vi "CString vs LStr Performance Comparison.vi"() -> ()   [LabVIEW 2020]
uses:
  <vilib>/Utility/file.llb/Application Directory.vi
  <vilib>/Utility/libraryn.llb/Check if File or Folder Exists.vi
panel:
  out "LStr Lossy Time":dbl
  out "LStr Lossy Results":i32[](array[numeric])
  out "CString Results":i32[](array[numeric])
  out "LStr Results":i32[](array[numeric])
  out "LStr Time":dbl
  out "CString Time":dbl
  # "This compares the performance between CStrings and LStr.\n\nAs expected LStr performance is better since it is the internal format.\n\nThis is aided by the speed of the encoding library vs the lossy from utf8."
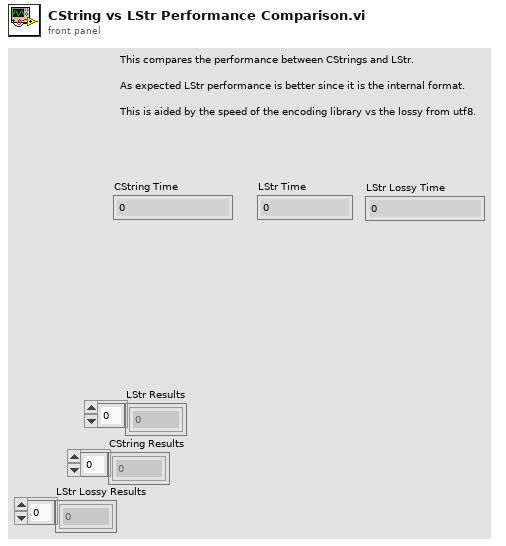
[diagram p1: front panel]
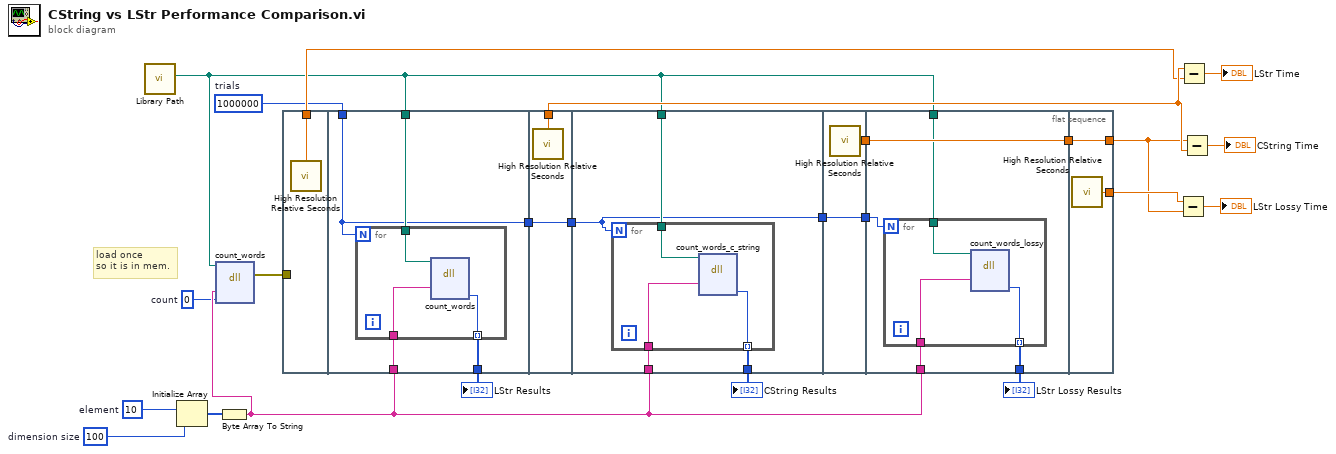
[diagram p0: block diagram]
diagram:
  w2 = 0  # count
  w14 = 100  # dimension size
  w15 = u8 10  # element
  w20 = 1000000  # trials
  # "load once\nso it is in mem."
  n1 = call "Library Path.vi"() -> ("Library Path"=w3:path)  [unwired: 11 in]
  n2 = Initialize Array(w15, w14) -> (w13:u8[])
  n3 = Byte Array To String(unsigned byte array=w13) -> (string=w4:string)
  n4 = dll-call lib="C:/Users/JamesMcNally/Documents/RustInterop/Rust-LabVIEW-Interop/target/debug/labview_test_library.dll" fn="count_words"(path in=w3, "string"=w4, "count"=w2) -> (error out=w1:errorcluster)  [unwired: 5 in, 1 out]
  n5 = flat-sequence {
    tunnel: [w25] -> w22
    tunnel: w1 -> [_]
    tunnel: w3 -> [w29]
    tunnel: w20 -> [w28]
    tunnel: [w28] -> w19
    tunnel: [w27] -> w17
    tunnel: w4 -> [w26]
    tunnel: [w34] -> w23
    tunnel: w19 -> [w33]
    tunnel: [w33] -> w18
    tunnel: w3 -> [w38]
    tunnel: w18 -> [w35]
    tunnel: [w37] -> w16
    tunnel: w4 -> [w36]
    tunnel: [w35] -> w6
    tunnel: [w43] -> w12
    tunnel: w6 -> [w42]
    tunnel: [w42] -> w5
    tunnel: w12 -> [w48]
    tunnel: w4 -> [w47]
    tunnel: w3 -> [w46]
    tunnel: [w45] -> w11
    tunnel: [w48] -> w10
    tunnel: w5 -> [w44]
    tunnel: [w53] -> w7
    tunnel: w10 -> [w53]
    tunnel: [w52] -> w8
    frame #0 {
      n6 = call <vilib>:"High Resolution Relative Seconds.vi"() -> ("relative seconds"=w25:dbl)
    }
    frame #1 {
      n7 = for {
        N: w28 -> [_]
        tunnel: w29 -> [w32]
        tunnel: [w31] -> w27 mode=indexing
        tunnel: w26 -> [w30]
        n8 = dll-call lib="C:/Users/JamesMcNally/Documents/RustInterop/Rust-LabVIEW-Interop/target/debug/labview_test_library.dll" fn="count_words"(path in=w32, "string"=w30) -> ("count"=w31:i32)  [unwired: 5 in, 2 out]
      }
    }
    frame #2 {
      n9 = call <vilib>:"High Resolution Relative Seconds.vi"() -> ("relative seconds"=w34:dbl)
    }
    frame #3 {
      n10 = for {
        N: w35 -> [_]
        tunnel: w38 -> [w41]
        tunnel: [w40] -> w37 mode=indexing
        tunnel: w36 -> [w39]
        n11 = dll-call lib="C:/Users/JamesMcNally/Documents/RustInterop/Rust-LabVIEW-Interop/target/debug/labview_test_library.dll" fn="count_words_c_string"(path in=w41, "string"=w39) -> ("count"=w40:i32)  [unwired: 5 in, 2 out]
      }
    }
    frame #4 {
      n12 = call <vilib>:"High Resolution Relative Seconds.vi"() -> ("relative seconds"=w43:dbl)
    }
    frame #5 {
      n13 = for {
        N: w44 -> [_]
        tunnel: w46 -> [w51]
        tunnel: [w50] -> w45 mode=indexing
        tunnel: w47 -> [w49]
        n14 = dll-call lib="C:/Users/JamesMcNally/Documents/RustInterop/Rust-LabVIEW-Interop/target/debug/labview_test_library.dll" fn="count_words_lossy"(path in=w51, "string"=w49) -> ("count"=w50:i32)  [unwired: 5 in, 2 out]
      }
    }
    frame #6 {
      n15 = call <vilib>:"High Resolution Relative Seconds.vi"() -> ("relative seconds"=w52:dbl)
    }
  }
  n16 = Subtract(x=w8, y=w7) -> (x-y=→"LStr Lossy Time":dbl)
  n17 = Subtract(x=w23, y=w22) -> (x-y=→"LStr Time":dbl)
  n18 = Subtract(x=w7, y=w23) -> (x-y=→"CString Time":dbl)
  "LStr Results" <- w17
  "CString Results" <- w16
  "LStr Lossy Results" <- w11
